vi "regresion.vi"() -> ()   [LabVIEW 2025]
uses:
  <vilib>/Analysis/Matrix/Datatypes/RealMatrix.ctl
  <vilib>/Analysis/baseanly.llb/Real A x B.vi
  <vilib>/Utility/file.llb/Read Delimited Spreadsheet (DBL).vi
  <vilib>/Analysis/Matrix/Numeric/Add/Add - RM,RM.vi
  <vilib>/Utility/file.llb/Read Delimited Spreadsheet (string).vi
  <vilib>/Analysis/NI_AALBase.lvlib
  <vilib>/Analysis/Matrix/NI_Matrix.lvlib
panel:
  out "A + B 2":T1
  out "all rows":string[][](array[string])
  out "期待される結果 2":dbl[][](array[numeric])
  out "入力 2":dbl[][](array[numeric])
  out "バイアス 2":dbl[][](array[numeric])
  out "重み 2":dbl[][](array[numeric])
  out "A + B":T1
  out "期待される結果":dbl[][](array[numeric])
  out "入力":dbl[][](array[numeric])
  out "バイアス":dbl[][](array[numeric])
  out "重み":dbl[][](array[numeric])
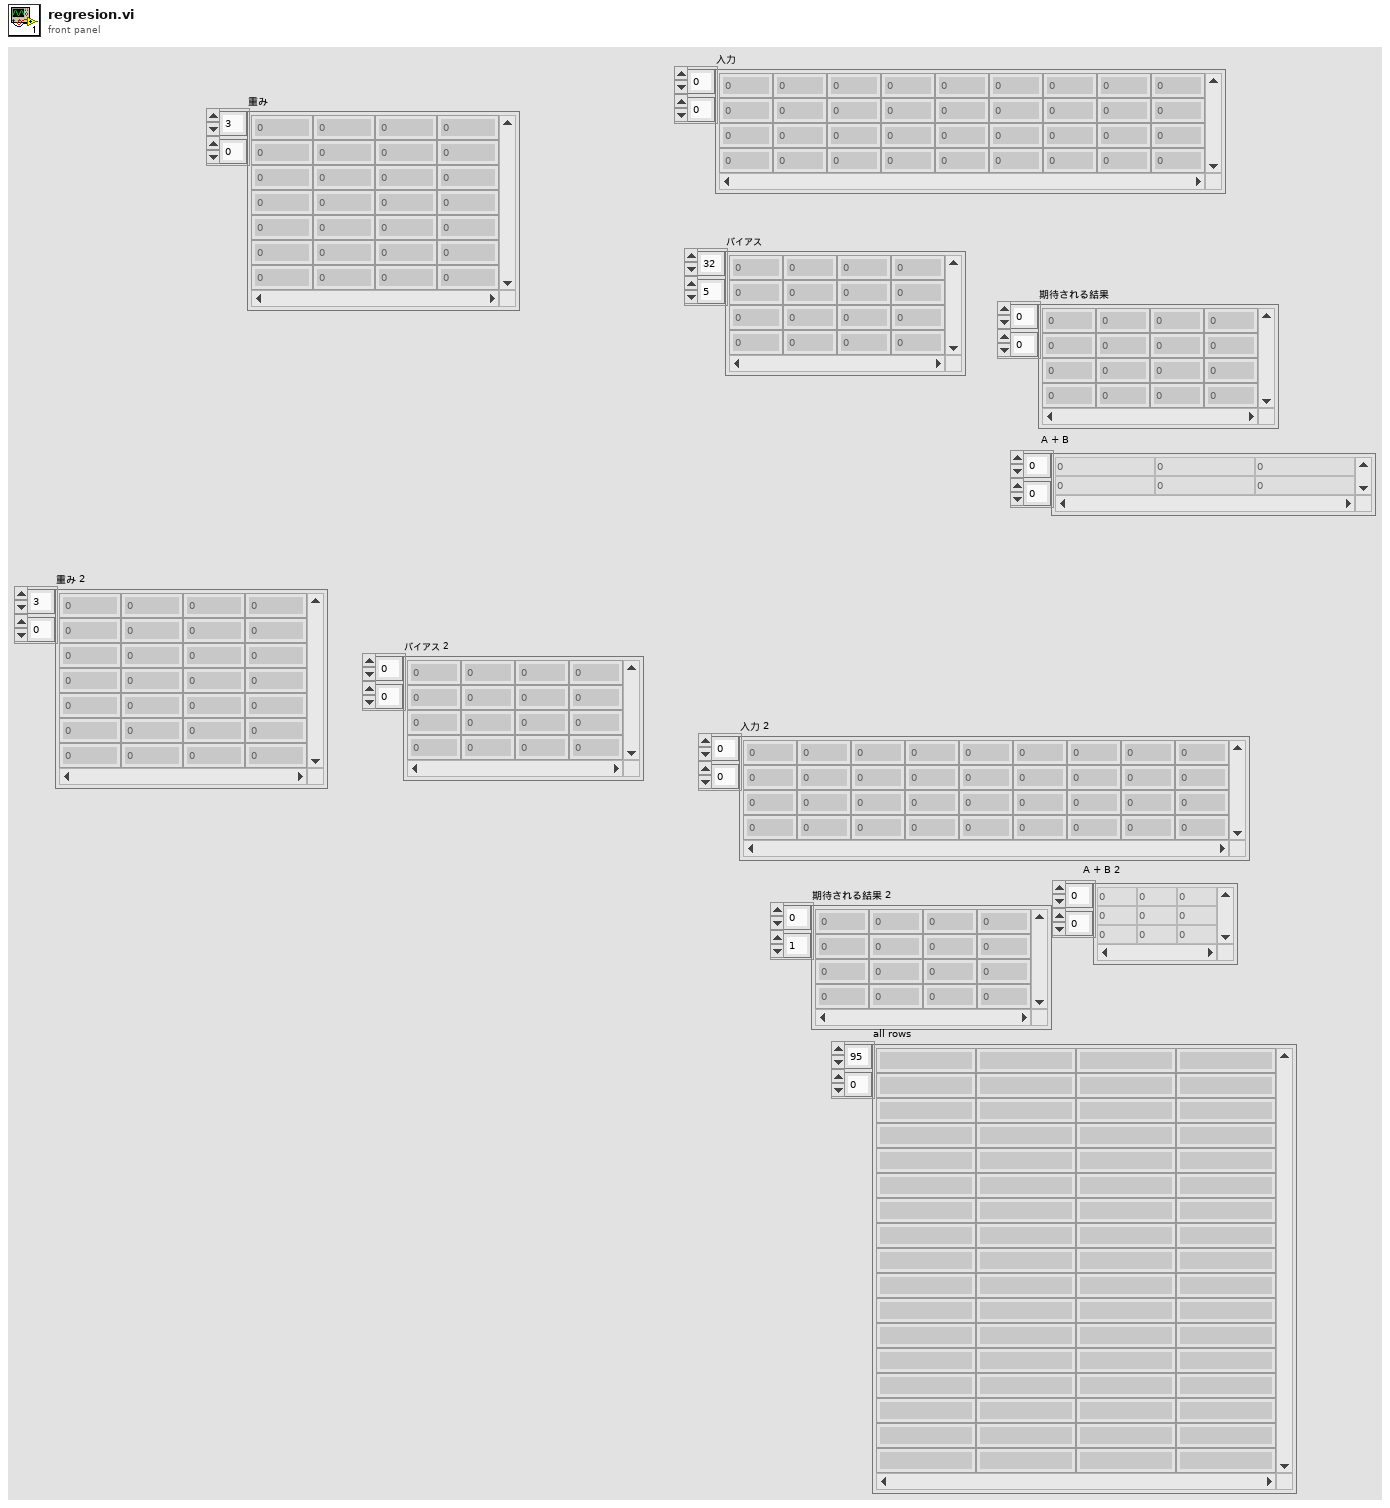
[diagram p1: front panel]
types:
  T1 = typedef "NI_Matrix.lvlib/RealMatrix.ctl" = dbl[][]
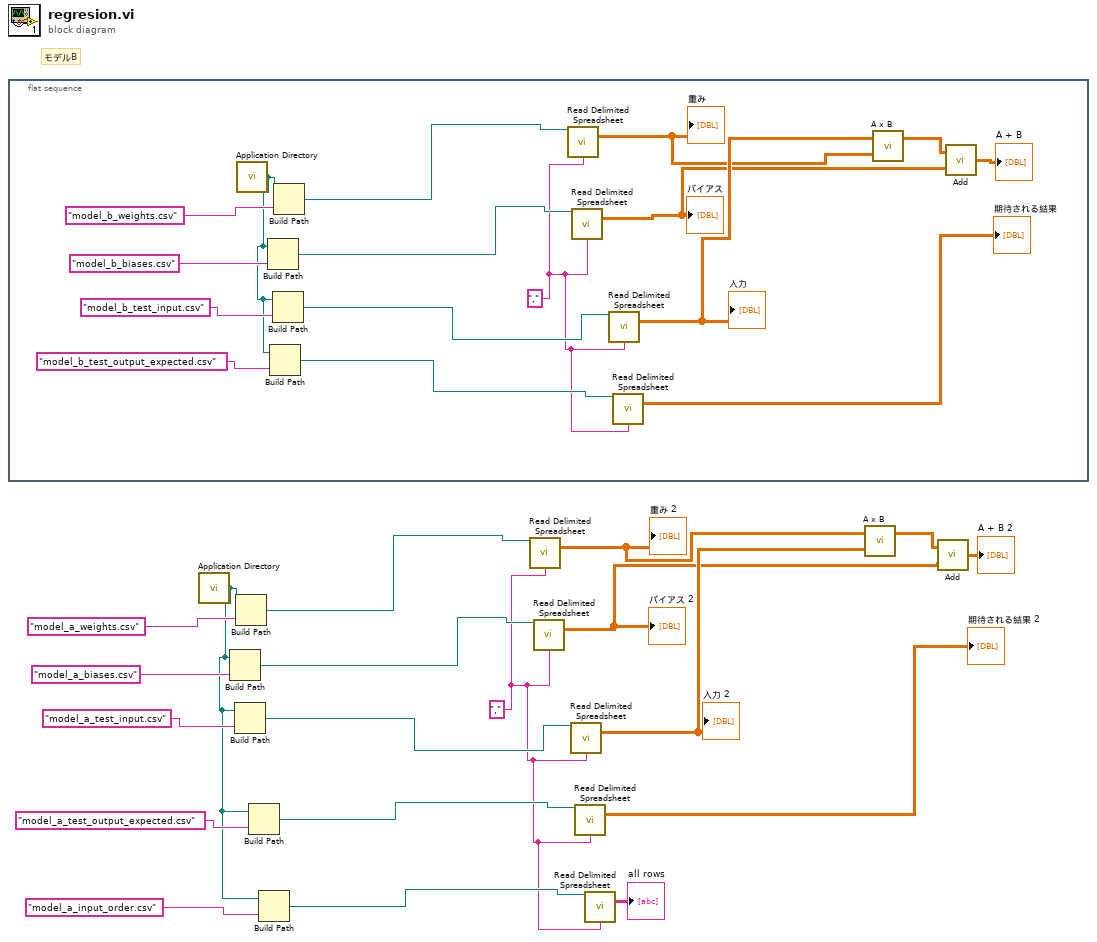
[diagram p0: block diagram]
diagram:
  w7 = ","
  # "モデルB"
  n1 = flat-sequence {
    frame #0 {
      w25 = ","
      n2 = call <vilib>:"Application Directory.vi"() -> ("Application Directory"=w30:path)
      n3 = Build Path(base path=w30, name or relative path="model_b_biases.csv") -> (appended path=w28:path)
      n4 = Build Path(base path=w30, name or relative path="model_b_test_output_expected.csv") -> (appended path=w26:path)
      n5 = Build Path(base path=w30, name or relative path="model_b_test_input.csv") -> (appended path=w27:path)
      n6 = Build Path(base path=w30, name or relative path="model_b_weights.csv") -> (appended path=w29:path)
      n7 = call-poly <vilib>:"Read Delimited Spreadsheet.vi"("file path (dialog if empty)"=w29, "delimiter (\\t)"=w25) -> ("all rows"=w23:dbl[][])  [unwired: 8 in, 5 out]
      "重み" <- w23
      n8 = call-poly <vilib>:"Read Delimited Spreadsheet.vi"("file path (dialog if empty)"=w28, "delimiter (\\t)"=w25) -> ("all rows"=w21:dbl[][])  [unwired: 8 in, 5 out]
      "バイアス" <- w21
      n9 = call-poly <vilib>:"Read Delimited Spreadsheet.vi"("file path (dialog if empty)"=w27, "delimiter (\\t)"=w25) -> ("all rows"=w24:dbl[][])  [unwired: 8 in, 5 out]
      "入力" <- w24
      n10 = call-poly <vilib>:"Read Delimited Spreadsheet.vi"("file path (dialog if empty)"=w26, "delimiter (\\t)"=w25) -> ("all rows"=→"期待される結果":dbl[][])  [unwired: 8 in, 5 out]
      n11 = call-poly <vilib>:"A x B.vi"("B"=w23, "A"=w24) -> ("A x B"=w22:T1)  [unwired: 1 out]
      n12 = call-poly <vilib>:"Add.vi"("Real Matrix B"=w21, "Real Matrix A"=w22) -> ("A + B"=→"A + B":T1)
    }
  }
  n13 = call <vilib>:"Application Directory.vi"() -> ("Application Directory"=w8:path)
  n14 = Build Path(base path=w8, name or relative path="model_a_biases.csv") -> (appended path=w13:path)
  n15 = Build Path(base path=w8, name or relative path="model_a_test_input.csv") -> (appended path=w12:path)
  n16 = Build Path(base path=w8, name or relative path="model_a_weights.csv") -> (appended path=w14:path)
  n17 = Build Path(base path=w8, name or relative path="model_a_test_output_expected.csv") -> (appended path=w11:path)
  n18 = Build Path(base path=w8, name or relative path="model_a_input_order.csv") -> (appended path=w9:path)
  n19 = call-poly <vilib>:"Read Delimited Spreadsheet.vi"("file path (dialog if empty)"=w14, "delimiter (\\t)"=w7) -> ("all rows"=w3:dbl[][])  [unwired: 8 in, 5 out]
  "重み 2" <- w3
  n20 = call-poly <vilib>:"Read Delimited Spreadsheet.vi"("file path (dialog if empty)"=w13, "delimiter (\\t)"=w7) -> ("all rows"=w2:dbl[][])  [unwired: 8 in, 5 out]
  "バイアス 2" <- w2
  n21 = call-poly <vilib>:"Read Delimited Spreadsheet.vi"("file path (dialog if empty)"=w12, "delimiter (\\t)"=w7) -> ("all rows"=w4:dbl[][])  [unwired: 8 in, 5 out]
  "入力 2" <- w4
  n22 = call-poly <vilib>:"Read Delimited Spreadsheet.vi"("file path (dialog if empty)"=w11, "delimiter (\\t)"=w7) -> ("all rows"=→"期待される結果 2":dbl[][])  [unwired: 8 in, 5 out]
  n23 = call-poly <vilib>:"Read Delimited Spreadsheet.vi"("file path (dialog if empty)"=w9, "delimiter (\\t)"=w7) -> ("all rows"=→"all rows":string[][])  [unwired: 8 in, 5 out]
  n24 = call-poly <vilib>:"A x B.vi"("B"=w4, "A"=w3) -> ("A x B"=w5:T1)  [unwired: 1 out]
  n25 = call-poly <vilib>:"Add.vi"("Real Matrix B"=w2, "Real Matrix A"=w5) -> ("A + B"=→"A + B 2":T1)
